vi "AtDome_logEvent_azimuthMovingDirection.vi"(8 "error in (no error)":errorcluster, 11 "logevent_azimuthMovingDirection_Ctl":T1) -> (0 "error out":errorcluster, 2 "function return":i32, 3 "logevent_azimuthMovingDirection_Ctl out":T1)   [LabVIEW 2016, in "SALLV_AtDome.lvlib"]
doc: "int AtDome_shm_logEvent_azimuthMovingDirectionLV(AtDome_logevent_azimuthMovingDirectionLV *logevent_azimuthMovingDirection_Ctl );"
uses:
  SALLV_AtDome.lvlib
  DataTypes/logevent_azimuthMovingDirection.ctl
  SALLV_AtDome.so
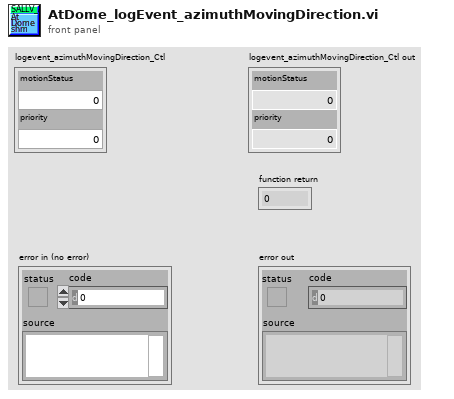
[diagram p1: front panel]
types:
  T1 = typedef "SALLV_AtDome.lvlib/logevent_azimuthMovingDirection.ctl" = cluster{"motionStatus":i32, "priority":i32}
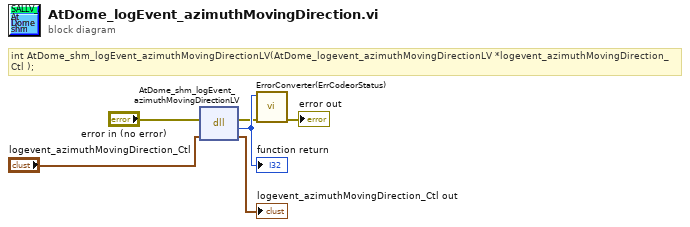
[diagram p0: block diagram]
diagram:
  # "int AtDome_shm_logEvent_azimuthMovingDirectionLV(AtDome_logevent_azimuthMovingDirectionLV *logevent_azimuthMovingDirection_Ctl );"
  n1 = dll-call lib="home/andres/Desktop/SAL_AtDome/SALLV_AtDome.*" fn="AtDome_shm_logEvent_azimuthMovingDirectionLV"(error in="error in (no error)", "logevent_azimuthMovingDirection_Ctl"="logevent_azimuthMovingDirection_Ctl") -> (error out=w2:errorcluster, w6:i32, "logevent_azimuthMovingDirection_Ctl"=→"logevent_azimuthMovingDirection_Ctl out":T1)  [unwired: 2 in, 1 out]
  "function return" <- w6
  n2 = call "ErrorConverter(ErrCodeorStatus).vi"("error in (no error)"=w2, "error code"=w6) -> ("error out"=→"error out":errorcluster)  [unwired: 9 in]
